vi "DataChosen.vi"(0 "Phasor Index":u16[](array[numeric]), 1 "Boolean array":bool[][](array[boolean]), 5 "PMU Number in List":u16[](array[numeric]), 7 "Phasor  Number in List":u16[](array[numeric]), 9 "Complex Phasors":csg[][](array[numeric]), 11 "Analog Values":sgl[][](array[numeric]), 12 "Frequency":sgl[](array[numeric]), 13 "dFreq":sgl[](array[numeric])) -> (4 "Complex Phasors Output":csg[](array[numeric]), 6 "FREQ Values":dbl[](array[numeric]), 8 "DFREQ Values":dbl[](array[numeric]))   [LabVIEW 2013]
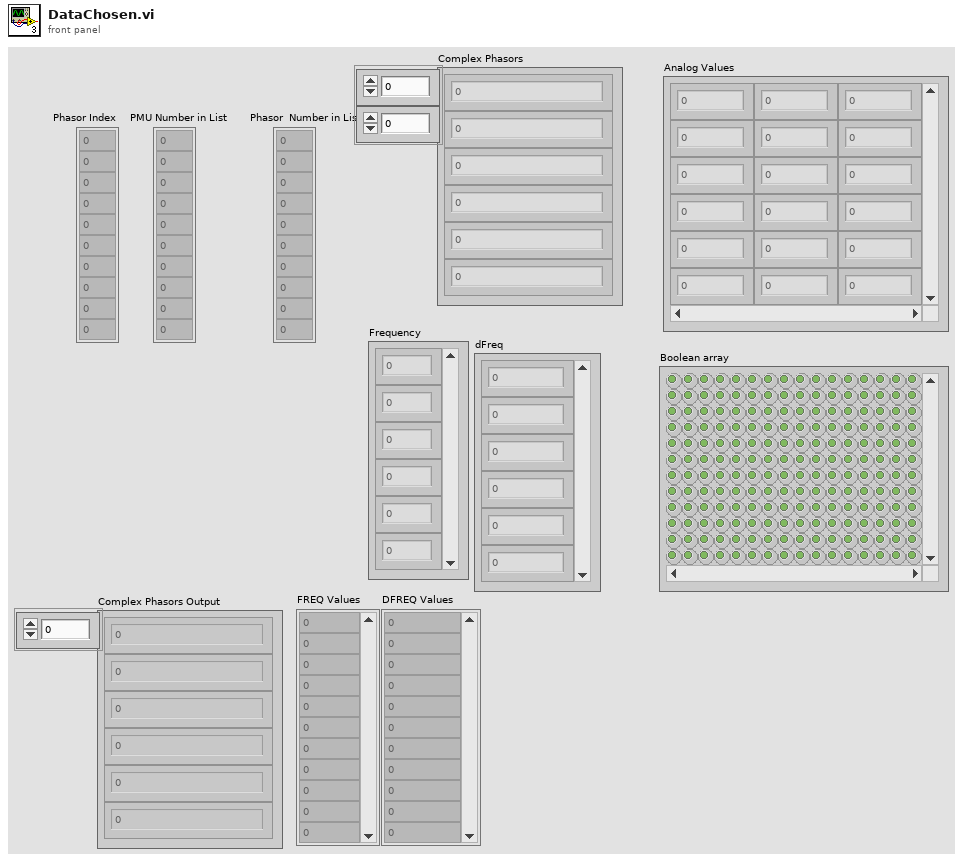
[diagram p1: front panel]
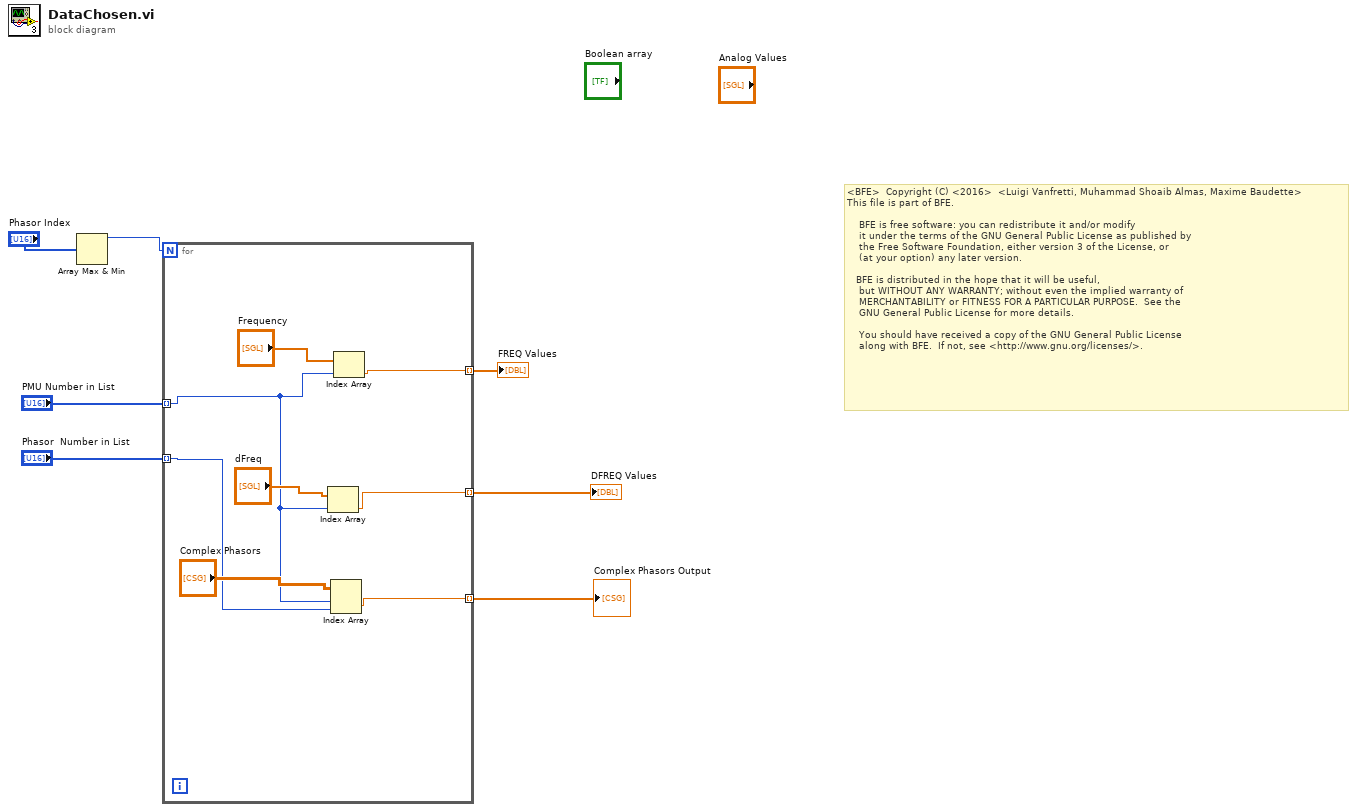
[diagram p0: block diagram]
diagram:
  # "<BFE>  Copyright (C) <2016>  <Luigi Vanfretti, Muhammad Shoaib Almas, Maxime Baudette> \nThis file is part of BFE.\n\n    BFE is free software: you can redistribute it and/or modify\n    it under the terms of the GNU General Public License as published by\n    the Free Software Foundation, either version 3 of the License, or\n    (at your option) any later version.\n\n   BFE is distributed in the hope that it will be useful,\n    but WITHOUT ANY WARRANTY; without even the implied warranty of\n    MERCHANTABILITY or FITNESS FOR A PARTICULAR PURPOSE.  See the\n    GNU General Public License for more details.\n\n    You should have received a copy of the GNU General Public License\n    along with BFE.  If not, see <http://www.gnu.org/licenses/>."
  n1 = Array Max & Min(array="Phasor Index") -> (max value=w7:u16)  [unwired: 3 out]
  n2 = for {
    N: w7 -> [_]
    tunnel: "PMU Number in List" -> [w12] mode=indexing
    tunnel: "Phasor  Number in List" -> [w11] mode=indexing
    tunnel: [w10] -> w3 mode=indexing
    tunnel: [w9] -> w2 mode=indexing
    tunnel: [w8] -> w1 mode=indexing
    n3 = Index Array(array="dFreq", index=w12) -> (element=w9:sgl)
    n4 = Index Array(array="Complex Phasors", index (row)=w12, index (col)=w11) -> (element=w8:csg)
    n5 = Index Array(array="Frequency", index=w12) -> (element=w10:sgl)
  }
  "DFREQ Values" <- w2
  "FREQ Values" <- w3
  "Complex Phasors Output" <- w1
